vi "更新程序.vi"() -> ()   [LabVIEW 2016, in "自动更新.lvlib"]
uses:
  <vilib>/FTP/NI_FTP.lvlib
panel:
  out "对比MD5":string
  out "当前MD5":string
  out "FTP链接结束":bool
  out "updateconfiguration":T1
  out "软件版本 2":string caption="目标软件版本"
  out "软件版本":string caption="当前软件版本"
  out "下载的文件名":string
  out "目标文件夹名":string
  out "端口号":i32
  out "IP地址":string
  out "步骤":string
  out "枚举":T2(ring)
  in  "目标路径（使用对话框）":path
  out "下载保存目录":path
  out "更新进度":u8(slide) scale=0.0..100.0
  # "1.下载更新--------2.MD5校验-------2.关闭主应用-------3.替换应用--------4.打开主应用-----------5.关闭本程序"
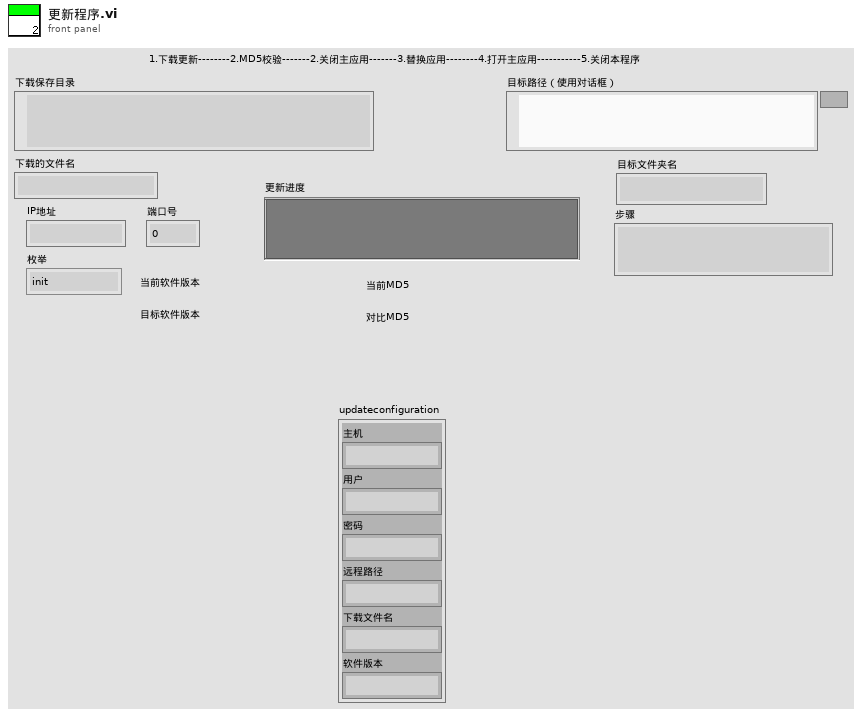
[diagram p1: front panel]
types:
  T1 = cluster{"主机":string, "用户":string, "密码":string, "远程路径":string, "下载文件名":string, "软件版本":string}
  T2 = enum16{"init", "download", "close", "replace", "open", "over"}
  T3 = typedef "NI_FTP.lvlib/FTP File Info.ctl" = cluster{"type":enum16{"unknown", "file", "dir", "link"}, "permissions":string, "owner":string, "group":string, "size":i32, "date":string, "name":string, "link name":string}
  T4 = enum16{"open", "replace", "create", "open or create", "replace or create", "replace or create with confirmation"}
  T5 = cluster{"网络灯":bool, "接收中":bool, "已接收百分比":u8, "接收成功次数":dbl, "当前步骤":enum16{"init", "receivehead", "receivecontent", "receivesuccess", "over"}, "文件名":string, "error out":errorcluster}
  T6 = cluster{"remote path":string, "local path":path, "binary":bool}
  T7 = typedef "NI_FTP.lvlib/FTP Session.ctl" = refnum<k5>
  T8 = cluster{"remote path":string, "local path":path, "binary":bool}[]
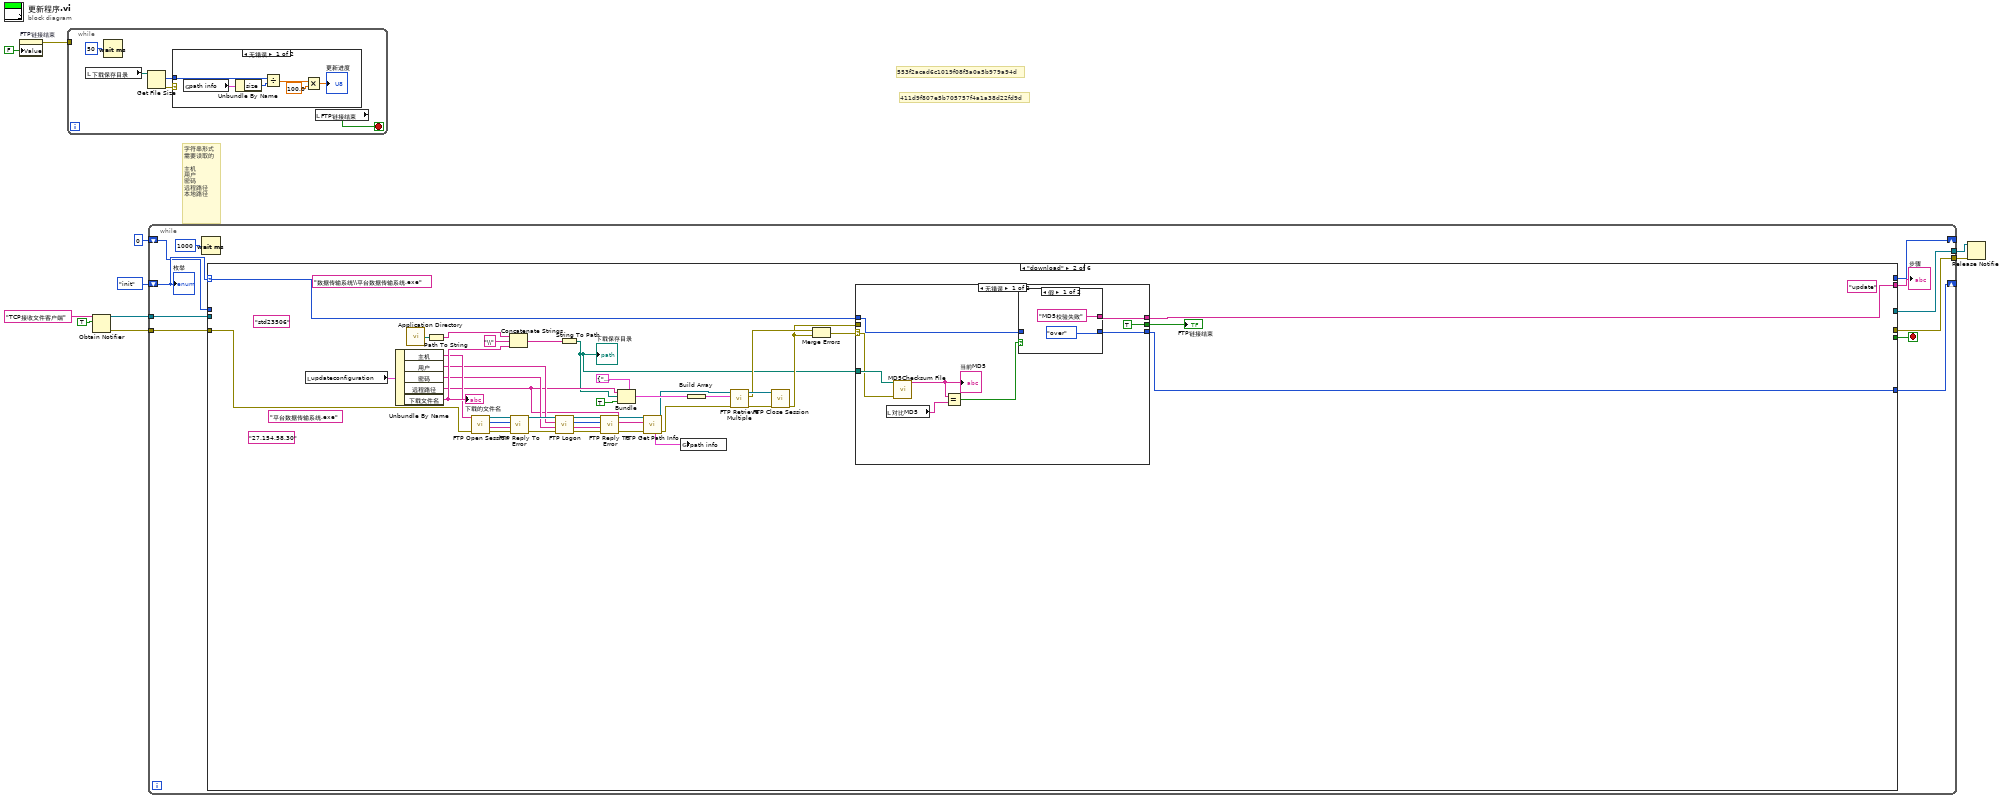
[diagram p0: block diagram]
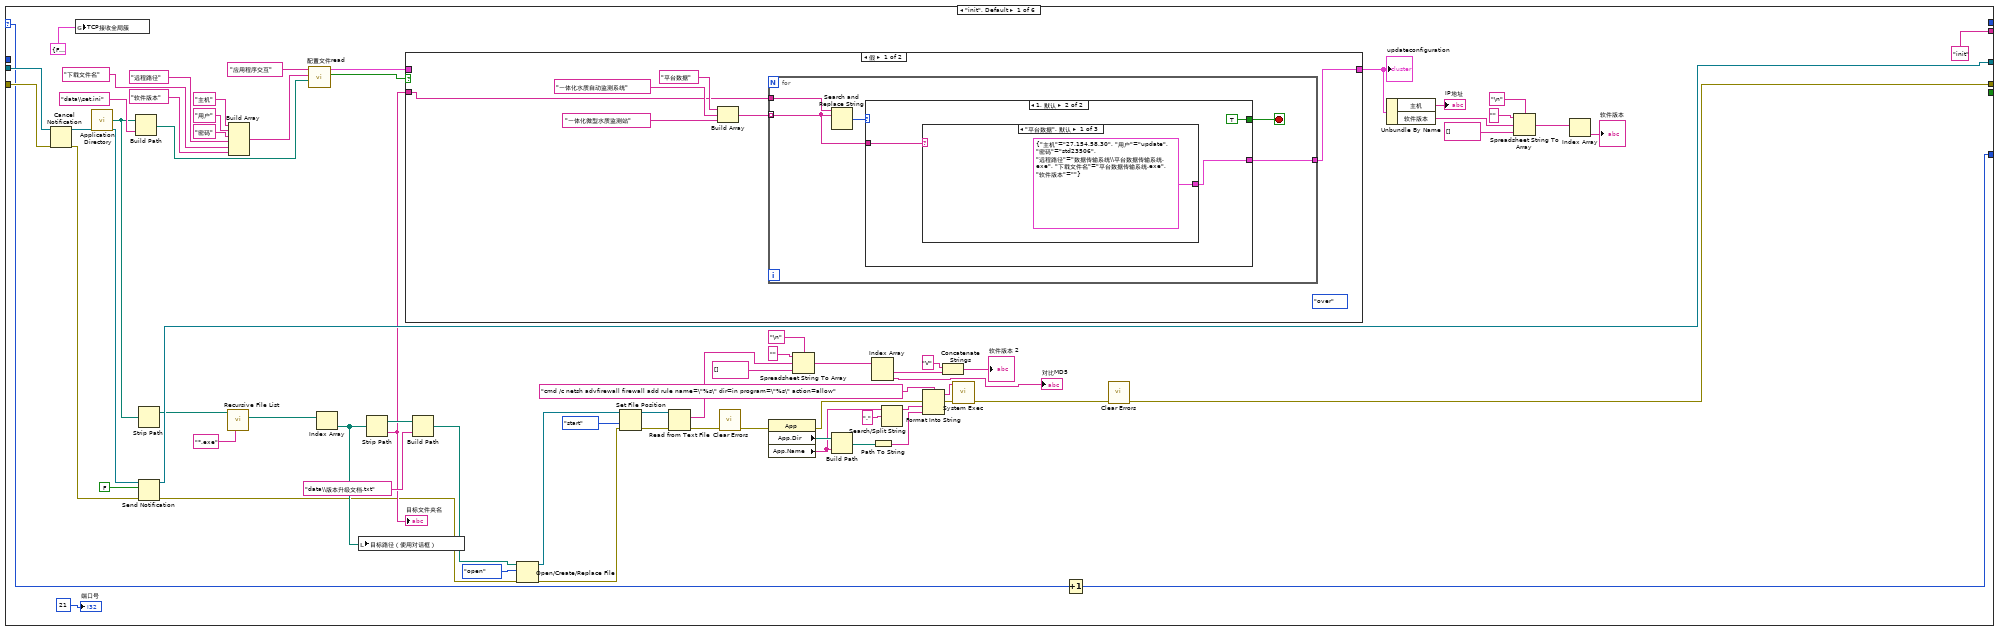
[diagram p3: hidden frame]
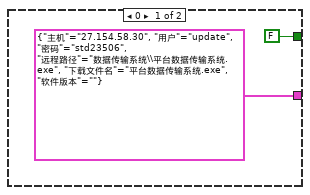
[diagram p4: hidden frame]
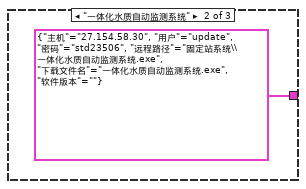
[diagram p5: hidden frame]
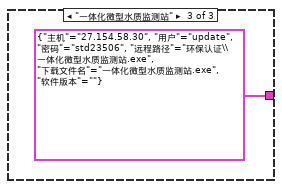
[diagram p6: hidden frame]
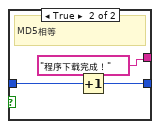
[diagram p8: hidden frame]
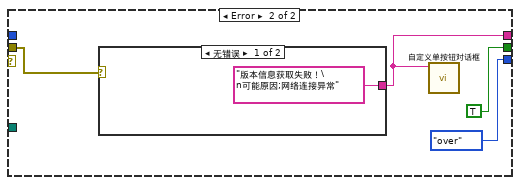
[diagram p9: hidden frame]
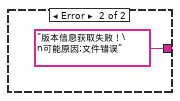
[diagram p10: hidden frame]
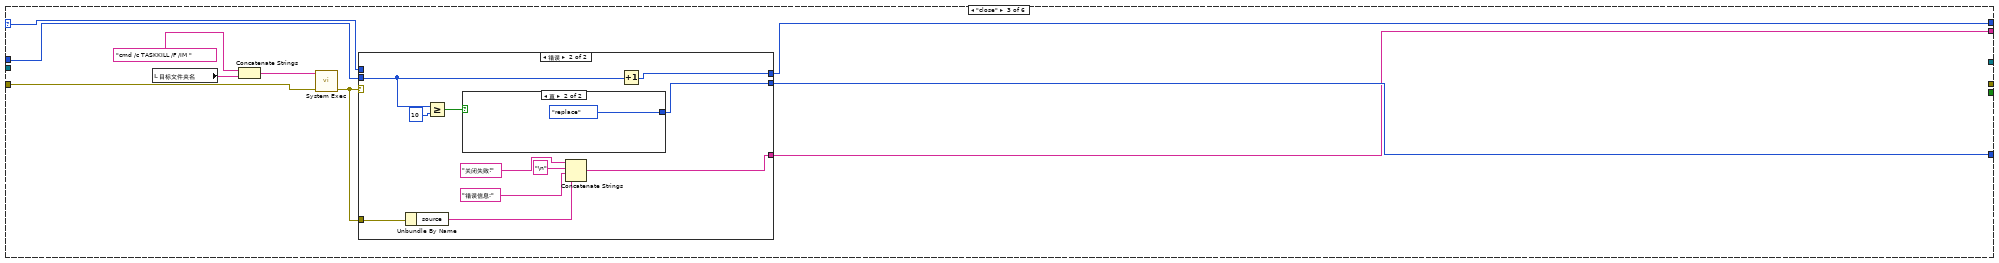
[diagram p11: hidden frame]
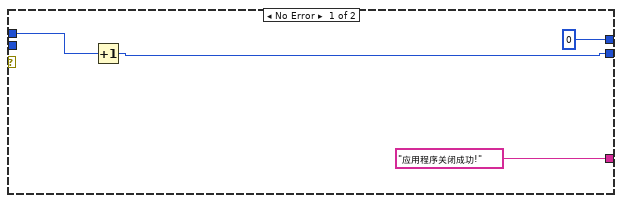
[diagram p12: hidden frame]
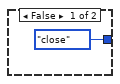
[diagram p13: hidden frame]
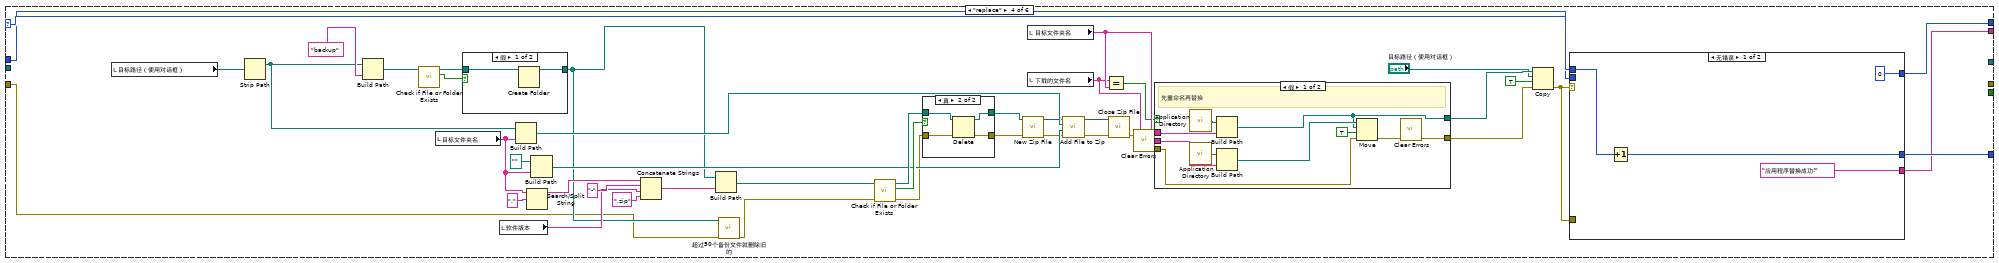
[diagram p14: hidden frame]
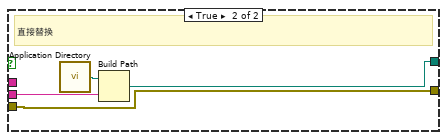
[diagram p17: hidden frame]
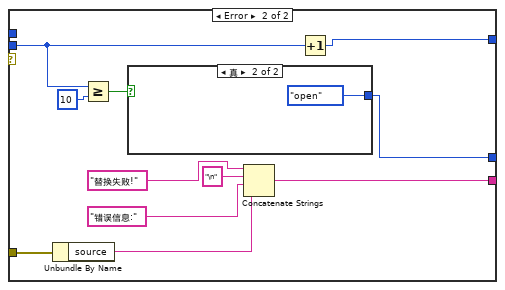
[diagram p18: hidden frame]
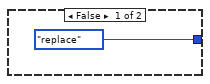
[diagram p19: hidden frame]
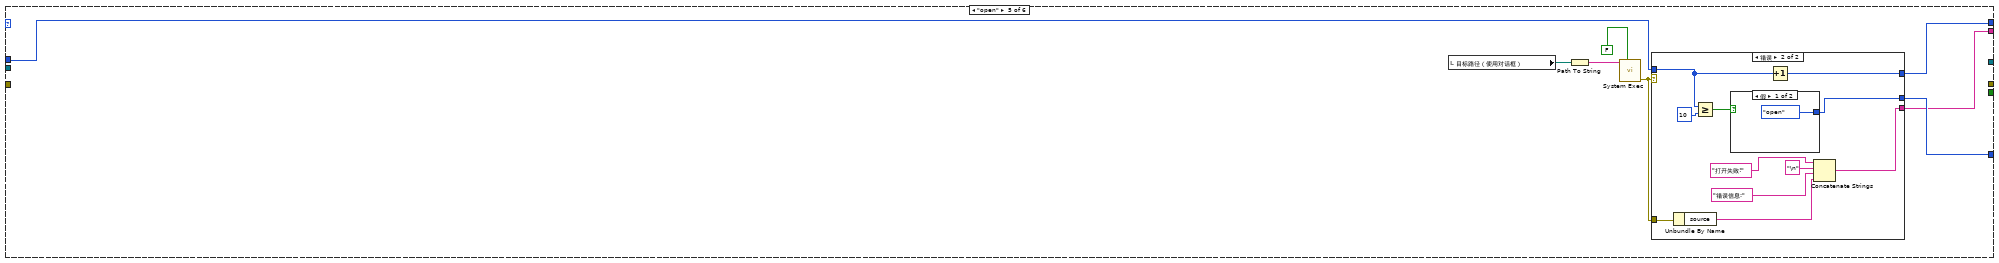
[diagram p20: hidden frame]
diagram:
  # "411d9f807e5b705757f4a1a38d22fd9d"
  # "553f2acad6c1019f08f3a0a5b979a94d"
  # "字符串形式\n需要读取的\n\n主机\n用户\n密码\n远程路径\n本地路径"
  n1 = property on="FTP链接结束" class="Bool (严格)"("Value"=FALSE ("FTP链接结束")) -> (error out=w1:errorcluster)  [unwired: 2 in, 1 out]
  n2 = while {
    tunnel: w1 -> [_]
    stop <- w15 stop-if-true
    n3 = local read "下载保存目录"() -> (w13:path)
    n4 = Wait (ms)(milliseconds to wait=u32 50 ("等待时间（毫秒）")) -> ()  [unwired: 1 out]
    n5 = Get File Size(file=w13) -> (size (in bytes)=w11:i64, 0:w12:errorcluster)  [unwired: 1 in, 1 out]
    n6 = case shown="无错误" w12 {
      tunnel: w11 -> [w17 _]
      frame No Error {
        n7 = global read "update全局.vi" "path info"() -> (w18:T3)
        n8 = Unbundle By Name(w18) -> ("size"=w21:i32)
        n9 = Divide(x=w17, y=w21) -> (x/y=w20:dbl)
        n10 = Multiply(x=w20, y=100.0) -> (x*y=→"更新进度":dbl)
      }
      frame Error {
      }
    }
    n11 = local read "FTP链接结束"() -> (w15:bool)
  }
  n12 = Obtain Notifier(name (unnamed)="TCP接收文件客户端" ("名称（未命名）"), notification data type=TRUE) -> (notifier out=w7:refnum<notifier>, error out=w6:errorcluster)  [unwired: 2 in, 1 out]
  n13 = while {
    shift-right: [w31] -> _
    shift-left: T2."init" -> [w32]
    tunnel: w7 -> [w27]
    tunnel: w6 -> [w26]
    tunnel: [w25] -> w5
    tunnel: [w24] -> w4
    shift-right: [w22] -> _
    shift-left: u8 0 -> [w23]
    stop <- w30 stop-if-true
    n14 = Wait (ms)(milliseconds to wait=u32 1000 ("等待时间（毫秒）")) -> ()  [unwired: 1 out]
    n15 = case shown="\"download\"" w32 {
      selector: w32 -> [w50 w160 w189 w253 _ w343]
      tunnel: [w49 w161 w188 w252 w297 w342] -> w31
      tunnel: [_ _ _ _ _ w338] -> w30
      tunnel: ["init" ("步骤") w159 w187 w251 w296 "over" ("步骤")] -> w28
      tunnel: w27 -> [w101 _ _ _ _ w340]
      tunnel: w26 -> [w100 w124 w183 w212 _ w318]
      tunnel: [w96 _ _ _ _ w339] -> w25
      tunnel: [w35 _ _ _ _ w323] -> w24
      tunnel: w23 -> [_ _ w185 w243 w294 _]
      tunnel: [_ _ w184 w242 w295 _] -> w22
      frame "init", Default {
        n16 = Cancel Notification(0:w101, 3:w100) -> (8:w99:refnum<notifier>, 11:w97:errorcluster)  [unwired: 1 out]
        n17 = global write "全局变量1.vi" "TCP接收全局簇"(T5 {"网络灯"=FALSE, "接收中"=FALSE, "已接收百分比"=0, "接收成功次数"=0.0, "当前步骤"=enum."init", "文件名"="", "error out"={"status"=FALSE, "code"=0, "source"=""}} ("TCP接收全局簇")) -> ()
        n18 = call <vilib>:"Application Directory.vi"() -> ("Application Directory"=w57:path)
        n19 = Build Path(base path=w57, name or relative path="data\\set.ini" ("名称或相对路径")) -> (appended path=w60:path)
        n20 = Strip Path(path=w57) -> (stripped path=w91:path)  [unwired: 1 out]
        n21 = Send Notification(notification=FALSE ("通知"), notifier=w99, error in (no error)=w97) -> (notifier out=w96:refnum<notifier>, error out=w36:errorcluster)
        n22 = call <vilib>:"Recursive File List.vi"("pattern"="*.exe", "Folder Path"=w91) -> ("All Files in Dir"=w93:path[])  [unwired: 5 in, 4 out]
        n23 = Build Array("主机" ("section"), "用户" ("section"), "密码" ("key"), "远程路径" ("key"), "下载文件名" ("key"), "软件版本" ("key")) -> (w64:string[])
        n24 = call "配置文件read.vi"("configuration file path"=w60, "键数组"=w64, "段"="应用程序交互" ("section")) -> ("section exists?"=w66:bool, "updateconfiguration"=w67:T1)  [unwired: 6 in, 1 out]
        n25 = Index Array(array=w93) -> (element=w94:path)  [unwired: 1 in]
        n26 = local write "目标路径（使用对话框）"(w94) -> ()
        n27 = Strip Path(path=w94) -> (stripped path=w68:path, name=w51:string)
        "目标文件夹名" <- w51
        n28 = case shown="假" w66 {
          tunnel: w67 -> [_ w122]
          tunnel: [w103 w122] -> w59
          tunnel: w51 -> [w104 _]
          frame False {
            (unwired) T2."over"
            n29 = Build Array("平台数据" ("搜索字符串"), "一体化水质自动监测系统" ("搜索字符串"), "一体化微型水质监测站" ("搜索字符串")) -> (w105:string[])
            n30 = for {
              tunnel: w105 -> [w110] mode=indexing
              tunnel: w104 -> [w111]
              tunnel: [w109] -> w103
              stop <- w112 stop-if-true
              n31 = Search and Replace String(input string=w111, search string=w110) -> (number of replacements=w113:i32)  [unwired: 6 in, 3 out]
              n32 = case shown="1, 默认" w113 {
                tunnel: [FALSE TRUE] -> w112
                tunnel: w110 -> [_ w117]
                tunnel: [T1 {"主机"="27.154.58.30", "用户"="update", "密码"="std23506", "远程路径"="数据传输系统\\平台数据传输系统.exe", "下载文件名"="平台数据传输系统.exe", "软件版本"=""} ("updateconfiguration") w116] -> w109
                frame 0 {
                }
                frame 1, Default {
                  n33 = case shown="\"平台数据\", 默认" w117 {
                    tunnel: [T1 {"主机"="27.154.58.30", "用户"="update", "密码"="std23506", "远程路径"="数据传输系统\\平台数据传输系统.exe", "下载文件名"="平台数据传输系统.exe", "软件版本"=""} ("updateconfiguration") T1 {"主机"="27.154.58.30", "用户"="update", "密码"="std23506", "远程路径"="固定站系统\\一体化水质自动监测系统.exe", "下载文件名"="一体化水质自动监测系统.exe", "软件版本"=""} ("updateconfiguration") T1 {"主机"="27.154.58.30", "用户"="update", "密码"="std23506", "远程路径"="环保认证\\一体化微型水质监测站.exe", "下载文件名"="一体化微型水质监测站.exe", "软件版本"=""} ("updateconfiguration")] -> w116
                    frame "平台数据", Default {
                    }
                    frame "一体化水质自动监测系统" {
                    }
                    frame "一体化微型水质监测站" {
                    }
                  }
                }
              }
            }
          }
          frame True {
          }
        }
        "updateconfiguration" <- w59
        n34 = Build Path(base path=w68, name or relative path="data\\版本升级文档.txt" ("名称或相对路径")) -> (appended path=w76:path)
        n35 = Open/Create/Replace File(file path (use dialog)=w76, error in=w36, operation (0:open)=T4."open" ("操作(0:open)")) -> (refnum out=w71:refnum<file>, error out=w72:errorcluster)  [unwired: 3 in, 1 out]
        n36 = Set File Position(refnum=w71, from (0:start)=enum16{"start", "end", "current"}."start" ("自（0:起始）"), error in=w72) -> (refnum out=w75:refnum<file>, error out=w73:errorcluster)  [unwired: 1 in]
        n37 = Read from Text File(file (use dialog)=w75, error in=w73) -> (text=w83:string, error out=w40:errorcluster)  [unwired: 2 in, 2 out]
        n38 = call <vilib>:"Clear Errors.vi"("error in (no error)"=w40) -> ("error out"=w34:errorcluster)  [unwired: 5 in, 1 out]
        n39 = property class="App"(error in=w34) -> (error out=w39:errorcluster, "App.Dir"=w48:path, "App.Name"=w43:string)  [unwired: 1 in, 1 out]
        n40 = Spreadsheet String To Array(delimiter (Tab)="\n" ("分隔符(Tab)"), format string="" ("格式字符串"), spreadsheet string=w83, array type (2D Dbl)=string[] []) -> (array=w80:string[])
        n41 = Build Path(base path=w48, name or relative path=w43) -> (appended path=w47:path)
        n42 = Index Array(array=w80) -> (element #1=w81:string, element #2=→"对比MD5":string)  [unwired: 2 in]
        n43 = Path To String(path=w47) -> (string=w45:string)
        n44 = Search/Split String(string=w43, search string/char (-)="." ("搜索字符串/字符(-)")) -> (substring before match=w42:string)  [unwired: 1 in, 2 out]
        n45 = Format Into String(format string="cmd /c netsh advfirewall firewall add rule name=\"%s\" dir=in program=\"%s\" action=allow" ("command line"), error in=w39, w42, w45) -> (resulting string=w41:string, error out=w38:errorcluster)  [unwired: 1 in]
        n46 = Concatenate Strings("V" ("字符串"), w81) -> (→"软件版本 2":string)
        n47 = call <vilib>:"System Exec.vi"("error in (no error)"=w38, "command line"=w41) -> ("error out"=w37:errorcluster)  [unwired: 6 in, 3 out]
        n48 = Increment(x=w50) -> (x+1=w49:T2)
        n49 = call <vilib>:"Clear Errors.vi"("error in (no error)"=w37) -> ("error out"=w35:errorcluster)  [unwired: 5 in, 1 out]
        n50 = Unbundle By Name(w59) -> ("主机"=→"IP地址":string, "软件版本"=w52:string)
        n51 = Spreadsheet String To Array(delimiter (Tab)="\n" ("分隔符(Tab)"), format string="" ("格式字符串"), spreadsheet string=w52, array type (2D Dbl)=string[] []) -> (array=w86:string[])
        n52 = Index Array(array=w86) -> (element=→"软件版本":string)  [unwired: 1 in]
        "端口号" <- 21 ("端口号")
      }
      frame "download" {
        (unwired) "平台数据传输系统.exe" ("字符串")
        (unwired) "std23506" ("password")
        (unwired) "update" ("user")
        (unwired) "数据传输系统\\平台数据传输系统.exe" ("remote path")
        (unwired) "27.154.58.30" ("host")
        n53 = local read "updateconfiguration"() -> (w155:T1)
        n54 = Unbundle By Name(w155) -> ("主机"=w140:string, "用户"=w139:string, "密码"=w138:string, "远程路径"=w135:string, "下载文件名"=w153:string)
        "下载的文件名" <- w153
        n55 = call <vilib>:"Application Directory.vi"() -> ("Application Directory"=w158:path)
        n56 = Path To String(path=w158) -> (string=w157:string)
        n57 = call <vilib>:"FTP Open Session.vi"("error in (no error)"=w124, "address"=w140) -> ("error out"=w142:errorcluster, "reply string"=w144:string, "reply code"=w143:i32, "ftp session"=w141:T7)  [unwired: 2 in, 4 out]
        n58 = Concatenate Strings(w157, "\\" ("字符串"), w153) -> (w156:string)
        n59 = call <vilib>:"FTP Reply To Error.vi"("error in (no error)"=w142, "reply string in"=w144, "reply code in"=w143, "ftp session"=w141) -> ("error out"=w145:errorcluster, "ftp session out"=w146:T7)  [unwired: 2 out]
        n60 = call <vilib>:"FTP Logon.vi"("error in (no error)"=w145, "password"=w138, "user"=w139, "ftp session"=w146) -> ("error out"=w147:errorcluster, "reply string"=w149:string, "reply code"=w150:i32, "ftp session out"=w148:T7)  [unwired: 4 out]
        n61 = String To Path(string=w156) -> (path=w123:path)
        "下载保存目录" <- w123
        n62 = call <vilib>:"FTP Reply To Error.vi"("error in (no error)"=w147, "reply string in"=w149, "reply code in"=w150, "ftp session"=w148) -> ("error out"=w152:errorcluster, "ftp session out"=w151:T7)  [unwired: 2 out]
        n63 = Bundle(cluster=T6 {"remote path"="", "local path"=path "", "binary"=FALSE} ("transfer spec"), "remote path"=w135, "local path"=w123, "binary"=TRUE) -> (w137:T6)
        n64 = call <vilib>:"FTP Get Path Info.vi"("error in (no error)"=w152, "remote path"=w135, "ftp session"=w151) -> ("error out"=w131:errorcluster, "ftp session out"=w133:T7, "path info"=w132:T3)  [unwired: 4 in, 2 out]
        n65 = global write "update全局.vi" "path info"(w132) -> ()
        n66 = Build Array(w137) -> (w130:T8)
        n67 = call <vilib>:"FTP Retrieve Multiple.vi"("error in (no error)"=w131, "file specifications"=w130, "ftp session"=w133) -> ("error out"=w128:errorcluster, "file errors"=w127:errorcluster[], "ftp session out"=w129:T7)  [unwired: 2 in, 4 out]
        n68 = call <vilib>:"FTP Close Session.vi"("error in (no error)"=w128, "ftp session"=w129) -> ("error out"=w126:errorcluster)  [unwired: 9 out]
        n69 = Merge Errors(w127, w126) -> (w162:errorcluster)
        n70 = case shown="无错误" w162 {
          selector: w162 -> [w166 _]
          tunnel: w126 -> [_ w180]
          tunnel: [w171 T2."over"] -> w161
          tunnel: w160 -> [w170 _]
          tunnel: [w169 w178] -> w159
          tunnel: [TRUE ("FTP链接结束") TRUE ("FTP链接结束")] -> w125
          tunnel: w123 -> [w167 _]
          frame No Error {
            n71 = local read "对比MD5"() -> (w164:string)
            n72 = call <vilib>:"MD5Checksum File.vi"("error in (no error)"=w166, "Path"=w167) -> ("MD5 message-digest"=w165:string)  [unwired: 8 in, 1 out]
            "当前MD5" <- w165
            n73 = Equal?(x=w165, y=w164) -> (x = y?=w163:bool)
            n74 = case shown="假" w163 {
              tunnel: [T2."over" w176] -> w171
              tunnel: w170 -> [_ w175]
              tunnel: ["MD5校验失败" "程序下载完成！"] -> w169
              frame False {
              }
              frame True {
                # "MD5相等"
                n75 = Increment(x=w175) -> (x+1=w176:T2)
              }
            }
          }
          frame Error {
            n76 = case shown="无错误" w180 {
              tunnel: ["版本信息获取失败！\n可能原因;网络连接异常" "版本信息获取失败！\n可能原因;文件错误"] -> w178
              frame No Error {
              }
              frame Error {
              }
            }
            n77 = call "自定义单按钮对话框.vi"("消息"=w178) -> ()  [unwired: 11 in]
          }
        }
        "FTP链接结束" <- w125
      }
      frame "close" {
        n78 = local read "目标文件夹名"() -> (w186:string)
        n79 = Concatenate Strings("cmd /c TASKKILL /F /IM " ("command line"), w186) -> (w190:string)
        n80 = call <vilib>:"System Exec.vi"("error in (no error)"=w183, "command line"=w190) -> ("error out"=w192:errorcluster)  [unwired: 6 in, 3 out]
        n81 = case shown="错误" w192 {
          tunnel: [w194 w201] -> w188
          tunnel: w192 -> [_ w207]
          tunnel: ["应用程序关闭成功!" ("步骤") w202] -> w187
          tunnel: w189 -> [w195 _]
          tunnel: w185 -> [_ w197]
          tunnel: [u8 0 w199] -> w184
          frame No Error {
            n82 = Increment(x=w195) -> (x+1=w194:T2)
          }
          frame Error {
            n83 = Unbundle By Name(w207) -> ("source"=w206:string)
            n84 = Greater Or Equal?(x=w197, y=u8 10) -> (x >= y?=w198:bool)
            n85 = case shown="真" w198 {
              tunnel: [T2."close" T2."replace"] -> w201
              frame False {
              }
              frame True {
              }
            }
            n86 = Concatenate Strings("关闭失败!" ("消息"), "\n" ("字符串"), "错误信息:" ("字符串"), w206) -> (w202:string)
            n87 = Increment(x=w197) -> (x+1=w199:u8)
          }
        }
      }
      frame "replace" {
        n88 = local read "目标路径（使用对话框）"() -> (w220:path)
        n89 = Strip Path(path=w220) -> (stripped path=w219:path)  [unwired: 1 out]
        n90 = Build Path(base path=w219, name or relative path="backup" ("名称或相对路径")) -> (appended path=w235:path)
        n91 = call <vilib>:"Check if File or Folder Exists.vi"("path"=w235) -> ("file or folder exists?"=w236:bool, "dup path"=w237:path)  [unwired: 8 in, 1 out]
        n92 = local read "目标文件夹名"() -> (w218:string)
        n93 = case shown="假" w236 {
          tunnel: w237 -> [w261 w262]
          tunnel: [w260 w262] -> w213
          frame False {
            n94 = Create Folder(path (use dialog)=w261) -> (created path=w260:path)  [unwired: 2 in, 2 out]
          }
          frame True {
          }
        }
        n95 = local read "软件版本"() -> (w221:string)
        n96 = Build Path(base path=w219, name or relative path=w218) -> (appended path=w232:path)
        n97 = Search/Split String(string=w218, search string/char (-)="." ("搜索字符串/字符(-)")) -> (substring before match=w226:string)  [unwired: 1 in, 2 out]
        n98 = Build Path(base path=path "" ("Relative Path from 1 to 2"), name or relative path=w218) -> (appended path=w234:path)
        n99 = Concatenate Strings(w226, "-" ("字符串"), w221, ".zip" ("字符串")) -> (w227:string)
        n100 = Build Path(base path=w213, name or relative path=w227) -> (appended path=w214:path)
        n101 = call "超过50个备份文件就删除旧的.vi"("error in (no error)"=w212, "Folder Path"=w213) -> ("error out"=w211:errorcluster)  [unwired: 9 in]
        n102 = call <vilib>:"Check if File or Folder Exists.vi"("error in (no error)"=w211, "path"=w214) -> ("error out"=w216:errorcluster, "file or folder exists?"=w239:bool, "dup path"=w238:path)  [unwired: 7 in]
        n103 = case shown="真" w239 {
          tunnel: w238 -> [w255 w259]
          tunnel: [w255 w258] -> w240
          tunnel: w216 -> [w254 w257]
          tunnel: [w254 w256] -> w215
          frame False {
          }
          frame True {
            n104 = Delete(path (use dialog)=w259, error in=w257) -> (deleted path=w258:path, error out=w256:errorcluster)  [unwired: 3 in, 1 out]
          }
        }
        n105 = call <vilib>:"New Zip File.vi"("error in (no error)"=w215, "target"=w240) -> ("error out"=w228:errorcluster, "zip file out"=w229:i64)  [unwired: 1 in, 3 out]
        n106 = local read "目标文件夹名"() -> (w247:string)
        n107 = local read "下载的文件名"() -> (w246:string)
        n108 = call <vilib>:"Add File to Zip.vi"("error in (no error)"=w228, "destination path in zip"=w234, "source file path"=w232, "zip file in"=w229) -> ("error out"=w231:errorcluster, "zip file out"=w230:i64)  [unwired: 6 in]
        n109 = Equal?(x=w246, y=w247) -> (x = y?=w245:bool)
        n110 = call <vilib>:"Close Zip File.vi"("error in (no error)"=w231, "zip file in"=w230) -> ("error out"=w217:errorcluster)  [unwired: 5 in]
        n111 = call <vilib>:"Clear Errors.vi"("error in (no error)"=w217) -> ("error out"=w210:errorcluster)  [unwired: 5 in, 1 out]
        n112 = case shown="假" w245 {
          tunnel: w246 -> [w269 w275]
          tunnel: w247 -> [w268 _]
          tunnel: [w267 w274] -> w250
          tunnel: [w264 w273] -> w241
          tunnel: w210 -> [w263 w273]
          frame False {
            # "先重命名再替换"
            n113 = call <vilib>:"Application Directory.vi"() -> ("Application Directory"=w271:path)
            n114 = call <vilib>:"Application Directory.vi"() -> ("Application Directory"=w270:path)
            n115 = Build Path(base path=w271, name or relative path=w268) -> (appended path=w267:path)
            n116 = Build Path(base path=w270, name or relative path=w269) -> (appended path=w272:path)
            n117 = Move(source path=w272, error in=w263, 9:TRUE ("覆盖(F)"), 10:w267) -> (error out=w265:errorcluster)  [unwired: 1 in, 2 out]
            n118 = call <vilib>:"Clear Errors.vi"("error in (no error)"=w265) -> ("error out"=w264:errorcluster)  [unwired: 5 in, 1 out]
          }
          frame True {
            # "直接替换"
            n119 = call <vilib>:"Application Directory.vi"() -> ("Application Directory"=w276:path)
            n120 = Build Path(base path=w276, name or relative path=w275) -> (appended path=w274:path)
          }
        }
        n121 = Copy(8:w241, 9:TRUE ("覆盖(F)"), 10:"目标路径（使用对话框）", 11:w250) -> (0:w244:errorcluster)  [unwired: 1 in, 2 out]
        n122 = case shown="无错误" w244 {
          tunnel: [w278 w285] -> w252
          tunnel: w244 -> [_ w291]
          tunnel: ["应用程序替换成功!" ("步骤") w286] -> w251
          tunnel: w253 -> [w279 _]
          tunnel: w243 -> [_ w283]
          tunnel: [u8 0 w281] -> w242
          frame No Error {
            n123 = Increment(x=w279) -> (x+1=w278:T2)
          }
          frame Error {
            n124 = Unbundle By Name(w291) -> ("source"=w290:string)
            n125 = Greater Or Equal?(x=w283, y=u8 10) -> (x >= y?=w282:bool)
            n126 = case shown="真" w282 {
              tunnel: [T2."replace" T2."open"] -> w285
              frame False {
              }
              frame True {
              }
            }
            n127 = Concatenate Strings("替换失败!" ("消息"), "\n" ("字符串"), "错误信息:" ("字符串"), w290) -> (w286:string)
            n128 = Increment(x=w283) -> (x+1=w281:u8)
          }
        }
      }
      frame "open" {
        n129 = local read "目标路径（使用对话框）"() -> (w298:path)
        n130 = Path To String(path=w298) -> (string=w301:string)
        n131 = call <vilib>:"System Exec.vi"("wait until completion? (T)"=FALSE, "command line"=w301) -> ("error out"=w299:errorcluster)  [unwired: 6 in, 3 out]
        n132 = case shown="错误" w299 {
          tunnel: [T2."over" w309] -> w297
          tunnel: w299 -> [_ w315]
          tunnel: ["应用程序打开成功!" ("步骤") w310] -> w296
          tunnel: w294 -> [_ w307]
          tunnel: [u8 0 w305] -> w295
          frame No Error {
          }
          frame Error {
            n133 = Unbundle By Name(w315) -> ("source"=w314:string)
            n134 = Greater Or Equal?(x=w307, y=u8 10) -> (x >= y?=w306:bool)
            n135 = case shown="假" w306 {
              tunnel: [T2."open" T2."over"] -> w309
              frame False {
              }
              frame True {
              }
            }
            n136 = Increment(x=w307) -> (x+1=w305:u8)
            n137 = Concatenate Strings("打开失败!" ("消息"), "\n" ("字符串"), "错误信息:" ("字符串"), w314) -> (w310:string)
          }
        }
      }
      frame "over" {
        w338 = TRUE
        n138 = local read "软件版本 2"() -> (w320:string)
        n139 = local read "软件版本"() -> (w322:string)
        n140 = Concatenate Strings("更新完成！\n更新前版本号:" ("字符串"), w322, "\r", "更新后版本号:", w320, "\r") -> (w336:string)
        n141 = Build Array(w336) -> (w335:string[])
        n142 = call <vilib>:"Application Directory.vi"() -> ("Application Directory"=w333:path)
        n143 = call "更新log记录.vi"("路径"=w333, "错误输入（无错误）"=w318, "logname"="版本更新log", "数组"=w335) -> ("错误输出"=w331:errorcluster)  [unwired: 7 in]
        n144 = call <vilib>:"Clear Errors.vi"("error in (no error)"=w331) -> ("error out"=w330:errorcluster)  [unwired: 5 in, 1 out]
        n145 = Increment(x=w343) -> (x+1=w342:T2)
        n146 = Send Notification(notification=w338, notifier=w340, error in (no error)=w330) -> (notifier out=w339:refnum<notifier>, error out=w326:errorcluster)
        n147 = Current VI's Path() -> (path=w328:path)
        n148 = Open VI Reference(vi path=w328, error in (no error)=w326) -> (vi reference=w327:refnum<vi>, error out=w329:errorcluster)  [unwired: 4 in]
        n149 = invoke class="VI" method="FP.Close"(reference=w327, error in=w329) -> (reference out=w324:refnum<vi>, error out=w325:errorcluster)  [unwired: 1 in, 1 out]
        n150 = Close Reference(reference=w324, error in (no error)=w325) -> (error out=w323:errorcluster)
      }
    }
    "步骤" <- w28
    "枚举" <- w32
  }
  n151 = Release Notifier(notifier=w5, error in (no error)=w4) -> ()  [unwired: 1 in, 3 out]
